vi "N9030B.vi"() -> ()   [LabVIEW 2017]
uses:
  <instrlib>/Keysight XSAn/Keysight XSAn.lvlib
panel:
  out "actual points":i32
  in  "resource string":refnum<visa-resource-name> caption="resource name"
  out "error out":errorcluster {"code" format="%.0x"}
  in  "Keysight N9030B":T1={"resolution bandwidth"=3.0, "video bandwidth"=3.0, "center frequency"=15000.0, "span"=5000.0, "option string"=""} {"span" format="%#_6p"; "center frequency" format="%#_6p"; "video bandwidth" format="%#_6p"; "resolution bandwidth" format="%#_6p"}
  out "amplitude":dbl[](array[numeric])
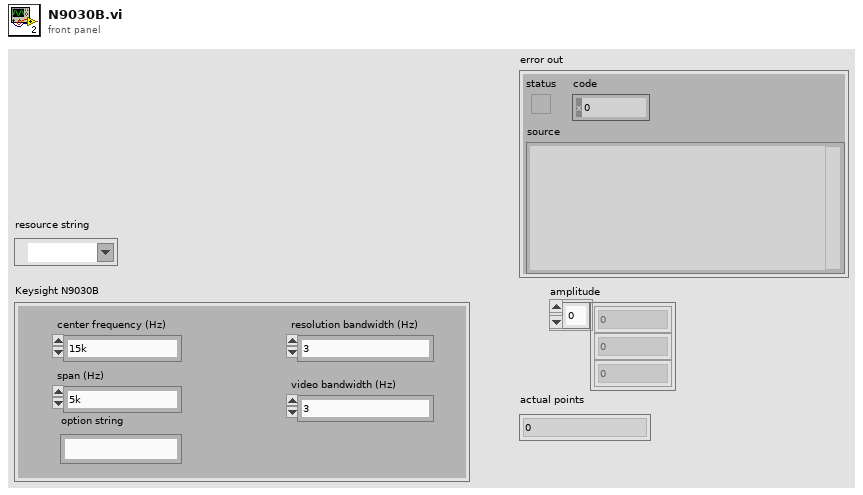
[diagram p1: front panel]
types:
  T1 = cluster{"resolution bandwidth":dbl, "video bandwidth":dbl, "center frequency":dbl, "span":dbl, "option string":string}
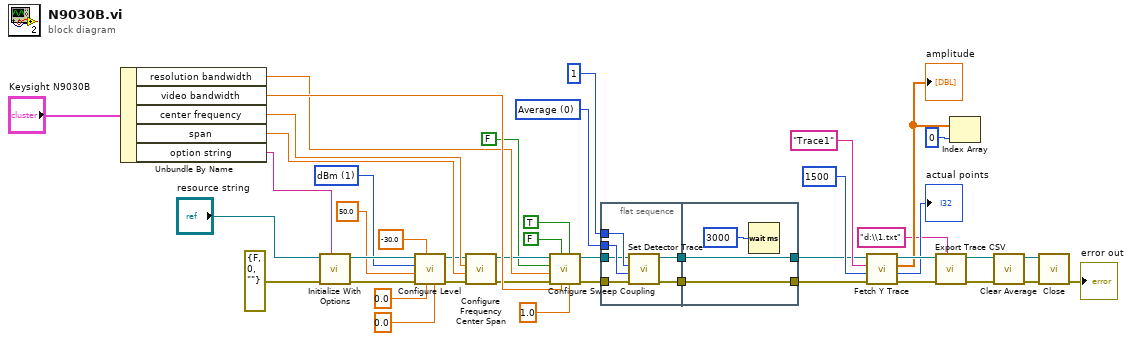
[diagram p0: block diagram]
diagram:
  w11 = 0 items=["Average", "Max Peak", "Min Peak", "Sample", "RMS", "Normal", "Quasi Peak", "EMI Average", "RMS Average", "Off"] ("DetectorType (Average)")
  w19 = 1 items=["dBm"=1, "dBmV"=2, "dBuV"=3, "Volt"=4, "Watt"=5] ("amplitude units (dBm)")
  n1 = Unbundle By Name("Keysight N9030B") -> ("resolution bandwidth"=w37:dbl, "video bandwidth"=w41:dbl, "center frequency"=w38:dbl, "span"=w39:dbl, "option string"=w40:string)
  n2 = call <instrlib>:"Initialize With Options.vi"("option string"=w40, "error in (no error)"=errorcluster {"status"=FALSE, "code"=0, "source"=""}, "resource string"="resource string") -> ("error out"=w22:errorcluster, "instrument handle out"=w23:refnum<k15>)  [unwired: 7 in]
  n3 = call <instrlib>:"Configure Level.vi"("attenuation"=0.0, "reference level offset"=0.0, "reference level"=-30.0, "error in (no error)"=w22, "input impedance"=50.0, "amplitude units (dBm)"=w19, "instrument handle"=w23) -> ("error out"=w26:errorcluster, "instrument handle out"=w25:refnum<k15>)  [unwired: 3 in]
  n4 = call <instrlib>:"Configure Frequency Center Span.vi"("error in (no error)"=w26, "span"=w39, "center frequency"=w38, "instrument handle"=w25) -> ("error out"=w33:errorcluster, "instrument handle out"=w32:refnum<k15>)  [unwired: 6 in]
  n5 = call <instrlib>:"Configure Sweep Coupling.vi"("sweep time"=1.0, "sweep time auto (Off)"=TRUE, "video bandwidth"=w41, "video bandwidth auto (Off)"=FALSE, "error in (no error)"=w33, "resolution bandwidth"=w37, "resolution bandwidth auto (Off)"=FALSE, "instrument handle"=w32) -> ("error out"=w10:errorcluster, "instrument handle out"=w9:refnum<k15>)  [unwired: 2 in]
  n6 = flat-sequence {
    tunnel: 1 ("TraceNo") -> [w50]
    tunnel: w11 -> [w49]
    tunnel: w10 -> [w48]
    tunnel: w9 -> [w47]
    tunnel: [w46] -> w44
    tunnel: [w45] -> w43
    tunnel: [w52] -> w7
    tunnel: [w53] -> w8
    tunnel: w44 -> [w53]
    tunnel: w43 -> [w52]
    frame #0 {
      n7 = call <instrlib>:"Set Detector Trace.vi"("error in (no error)"=w48, "DetectorType (Average)"=w49, "TraceNo"=w50, "instrument handle"=w47) -> ("error out"=w45:errorcluster, "instrument handle out"=w46:refnum<k15>)  [unwired: 6 in]
    }
    frame #1 {
      n8 = Wait (ms)(milliseconds to wait=u32 3000) -> ()  [unwired: 1 out]
    }
  }
  n9 = call <instrlib>:"Fetch Y Trace.vi"("error in (no error)"=w7, "array length"=1500, "trace name"="Trace1", "instrument handle"=w8) -> ("error out"=w35:errorcluster, "actual points"=→"actual points":i32, "amplitude"=w28:dbl[], "instrument handle out"=w34:refnum<k15>)  [unwired: 4 in]
  "amplitude" <- w28
  n10 = call <instrlib>:"Export Trace CSV.vi"("Filename"="d:\\1.txt" ("string"), "error in (no error)"=w35, "instrument handle"=w34) -> ("error out"=w4:errorcluster, "instrument handle out"=w5:refnum<k15>)  [unwired: 7 in]
  n11 = Index Array(array=w28, index=0) -> ()  [unwired: 1 out]
  n12 = call <instrlib>:"Clear Average.vi"("error in (no error)"=w4, "instrument handle"=w5) -> ("error out"=w2:errorcluster, "instrument handle out"=w3:refnum<k15>)  [unwired: 8 in]
  n13 = call <instrlib>:"Close.vi"("error in (no error)"=w2, "instrument handle"=w3) -> ("error out"=→"error out":errorcluster)  [unwired: 9 in]
